vi "re-count objects (SubVI).vi"(11 "output array in in":string[][](array[string])) -> (3 "output array out":string[][](array[string]))   [LabVIEW 2020]
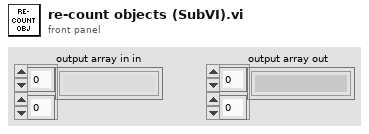
[diagram p1: front panel]
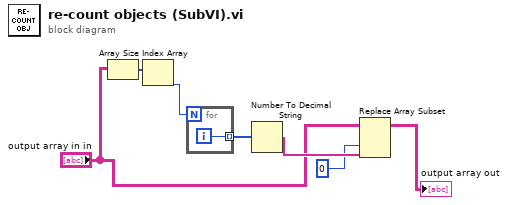
[diagram p0: block diagram]
diagram:
  n1 = Array Size(array="output array in in") -> (size(s)=w1:i32[])
  n2 = Index Array(array=w1) -> (element=w3:i32)  [unwired: 1 in]
  n3 = for {
    N: w3 -> [_]
    tunnel: [w8] -> w2 mode=indexing
    i -> [w8]
  }
  n4 = Number To Decimal String(number=w2) -> (decimal integer string=w6:string[])  [unwired: 1 in]
  n5 = Replace Array Subset(array="output array in in", new element=w6, index (col)=0 ("disabled index (col)")) -> (→"output array out":string[][])  [unwired: 1 in]
